vi "Wait on VI Idle.vi"(8 "error in (no error)":errorcluster, 9 "ms Polling Rate (1 ms)":u32=1, 10 "ms Timout (100ms)":u32=100, 11 "VI to Wait on":refnum<vi>) -> (0 "error out":errorcluster, 2 "Timeout?":bool, 3 "VI to Wait on dup":refnum<vi>)   [LabVIEW 2021, in "smo.lvlib" / "SMO.lvclass"]
doc: "Waits until the VIs specified by \"VIs to Wait on\" are unloaded from memory or a timeout occurs."
uses:
  SMO.lvclass
  SMO.lvclass/SMO.ctl
panel:
  # "Wait on VIs Unloaded from Memory.vi\n\nWaits until the VIs specified by \"VIs to Wait on\" are unloaded from memory or a timeout occurs.\n\nPlease visit http://www.OpenG.org to learn about the\nOpen Source LabVIEW software movement.\n\nNOTICE -- YOU MUST LEAVE THIS NOTICE IN PLACE.  PER THE TERMS OF THE LICENSE BELOW, YOU MAY SUBLICENSE THIS SOFTWARE \nIN ANY WAY THAT DOES NOT CONFLICT WITH THIS LICENSE.\n\n### BSD License (http://www.opensource.org/licenses/bsd-license.php) Begin ###\n \nCopyright (c) 2002, Jim Kring <jim@jimkring.com>\n\nAll rights reserved.\n\nRedistribution and use in source and binary forms, with or without modification, are permitted provided that the following conditions are met:\n\n    * Redistributions of source code must retain the above copyright notice, this list of conditions and the following disclaimer.\n    * Redistributions in binary form must reproduce the above copyright notice, this list of conditions and the following disclaimer in the \n       documentation and/or other materials provided with the distribution.\n    * Neither the name of SciWare, James Kring, Inc., nor the names of its contributors may be used to endorse or promote products derived \n       from this software without specific prior written permission.\n\nTHIS SOFTWARE IS PROVIDED BY THE COPYRIGHT HOLDERS AND CONTRIBUTORS \"AS IS\" AND ANY EXPRESS OR IMPLIED WARRANTIES, \nINCLUDING, BUT NOT LIMITED TO, THE IMPLIED WARRANTIES OF MERCHANTABILITY AND FITNESS FOR A PARTICULAR PURPOSE ARE \nDISCLAIMED. IN NO EVENT SHALL THE COPYRIGHT OWNER OR CONTRIBUTORS BE LIABLE FOR ANY DIRECT, INDIRECT, INCIDENTAL,\n SPECIAL, EXEMPLARY, OR CONSEQUENTIAL DAMAGES (INCLUDING, BUT NOT LIMITED TO, PROCUREMENT OF SUBSTITUTE GOODS OR \nSERVICES; LOSS OF USE, DATA, OR PROFITS; OR BUSINESS INTERRUPTION) HOWEVER CAUSED AND ON ANY THEORY OF LIABILITY, \nWHETHER IN CONTRACT, STRICT LIABILITY, OR TORT (INCLUDING NEGLIGENCE OR OTHERWISE) ARISING IN ANY WAY OUT OF THE USE \nOF THIS SOFTWARE, EVEN IF ADVISED OF THE POSSIBILITY OF SUCH DAMAGE.\n\n### BSD License End ###"
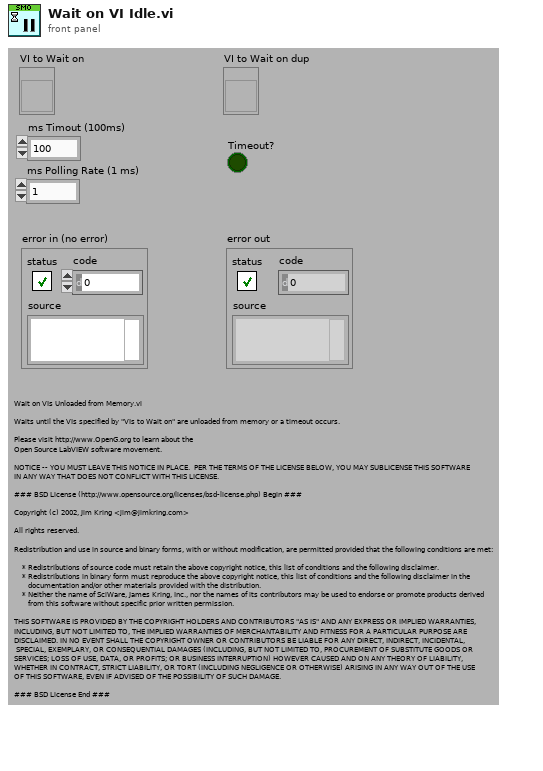
[diagram p1: front panel]
types:
  T1 = enum32{"Bad", "Idle", "Run top level", "Running"}
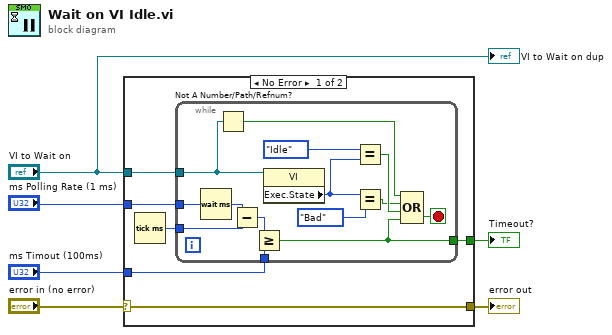
[diagram p0: block diagram]
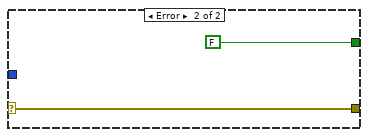
[diagram p2: hidden frame]
diagram:
  n1 = case shown="No Error" "error in (no error)" {
    selector: "error in (no error)" -> [w8 w28]
    tunnel: "VI to Wait on" -> [w12 _]
    tunnel: "ms Timout (100ms)" -> [w10 _]
    tunnel: [w9 FALSE] -> w5
    tunnel: [w8 w28] -> w3
    tunnel: "ms Polling Rate (1 ms)" -> [w7 _]
    frame No Error {
      n2 = Tick Count (ms)() -> (millisecond timer value=w11:u32)
      n3 = while {
        tunnel: w7 -> [w20]
        tunnel: [w21] -> w9
        tunnel: w10 -> [w23]
        tunnel: w11 -> [w25]
        tunnel: w12 -> [w18]
        stop <- w22 stop-if-true
        n4 = Wait (ms)(milliseconds to wait=w20) -> (millisecond timer value=w26:u32)
        n5 = Not A Number/Path/Refnum?(number/path/refnum=w18) -> (NaN/Path/Refnum?=w17:bool)
        n6 = Subtract(x=w26, y=w25) -> (x-y=w24:u32)
        n7 = Greater Or Equal?(x=w24, y=w23) -> (x >= y?=w21:bool)
        n8 = property class="VI"(reference=w18) -> ("Exec.State"=w15:T1)  [unwired: 1 in, 2 out]
        n9 = Equal?(x=T1."Idle", y=w15) -> (x = y?=w16:bool)
        n10 = Equal?(x=w15, y=T1."Bad") -> (x = y?=w13:bool)
        n11 = Compound Arithmetic op=OR(w17, w13, w16, w21) -> (w22:bool)
      }
    }
    frame Error {
    }
  }
  "Timeout?" <- w5
  "error out" <- w3
  "VI to Wait on dup" <- "VI to Wait on"
